vi "Check if configuration files exist.vi"(8 "error in (no error)":errorcluster, 11 "CascadeBase in":refnum<class "Cascade.lvclass">) -> (0 "error out":errorcluster, 2 "configuration file exists?":bool, 3 "CascadeBase out":refnum<class "Cascade.lvclass">)   [LabVIEW 2012, in "Cascade.lvclass"]
doc: "Checks whether all required configuration files for the component exist."
uses:
  Cascade.lvclass
  <vilib>/Distrio/Murmex/Murmex/Murmex.lvclass
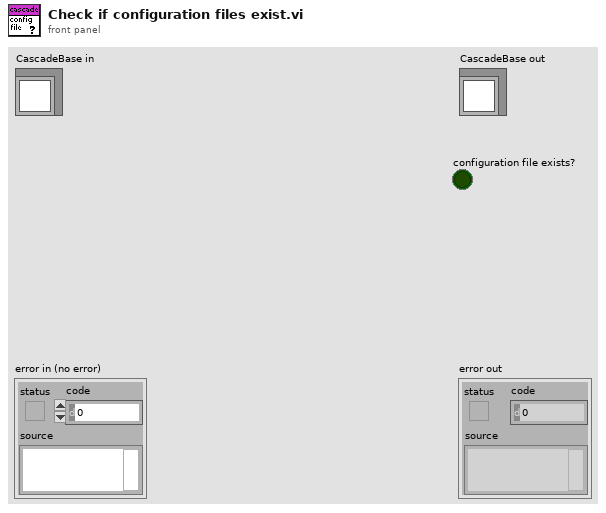
[diagram p1: front panel]
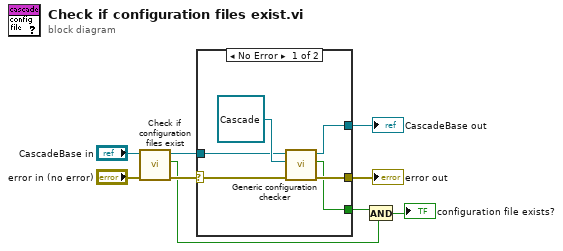
[diagram p0: block diagram]
diagram:
  n1 = call-parent "Check if configuration files exist.vi"("error in (no error)"="error in (no error)", "MurmexBase in"="CascadeBase in") -> ("error out"=w7:errorcluster, "configuration file exists?"=w1:bool, "MurmexBase out"=w5:refnum<class "Cascade.lvclass">)  [unwired: 7 in]
  n2 = case shown="No Error" w7 {
    selector: w7 -> [w15 w16]
    tunnel: [w14 w16] -> w6
    tunnel: w5 -> [w12 w17]
    tunnel: [w11 w17] -> w4
    tunnel: [w10 _] -> w2
    frame No Error {
      n3 = call <vilib>:"Generic configuration checker.vi"("error in (no error)"=w15, "inheritance level"=refnum<class "Cascade.lvclass"> refnum ("Cascade.lvclass"), "Murmex in"=w12) -> ("error out"=w14:errorcluster, "configuration file exists?"=w10:bool, "Murmex out"=w11:refnum<class "Cascade.lvclass">)  [unwired: 6 in]
    }
    frame Error {
    }
  }
  "error out" <- w6
  "CascadeBase out" <- w4
  n4 = And(x=w2, y=w1) -> (x .and. y?=→"configuration file exists?":bool)
